vi "DTtoASCII 3.vi"(1 "DutyCycle":dbl) -> (0 "String":string)   [LabVIEW 2014]
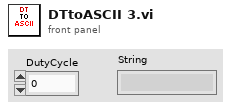
[diagram p1: front panel]
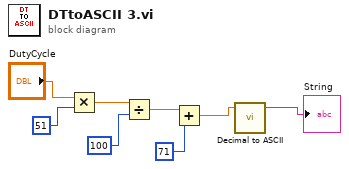
[diagram p0: block diagram]
diagram:
  n1 = Multiply(x="DutyCycle", y=51) -> (x*y=w6:dbl)
  n2 = Divide(x=w6, y=100) -> (x/y=w4:dbl)
  n3 = Add(x=w4, y=71) -> (x+y=w2:dbl)
  n4 = call "Decimal to ASCII.vi"("Decimal Number"=w2) -> ("Decimal String"=→"String":string)  [unwired: 2 in, 2 out]
